vi "Configure Sweep.vi"(0 "VISA resource name":refnum<visa-resource-name>, 1 "Source Type (1: Fixed)":i32(ring)=1 items=["Arbitrary", "Fixed", "Sweep", "List"], 2 "Sweep Output Type (0: Linear Single)":i32(ring) items=["Linear Single", "Linear Double"], 5 "Channel (1: Channel 1)":i32(ring)=1 items=["Channel 1"=1, "Channel 2"=2], 7 "Sweep Stop (0 V)":dbl, 9 "Sweep Start (0 V)":dbl, 11 "error in (no error)":errorcluster, 12 "Sweep Step Number (1)":i32=1) -> (4 "VISA resource name out":refnum<visa-resource-name>, 15 "error out":errorcluster)   [LabVIEW 2012, in "Keysight B2980 Series.lvlib"]
doc: "Configures sweep for measurement and source.\n\n<b>Note(s):</b>\nThis VI is only applicable for model B2985A and B2987A."
uses:
  Keysight B2980 Series.lvlib
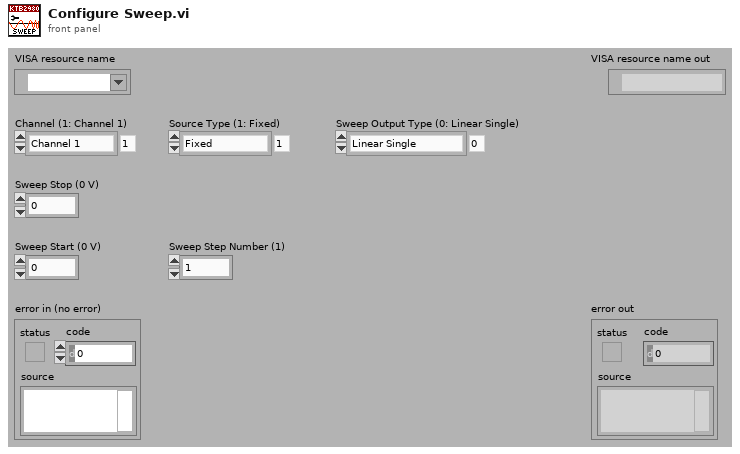
[diagram p1: front panel]
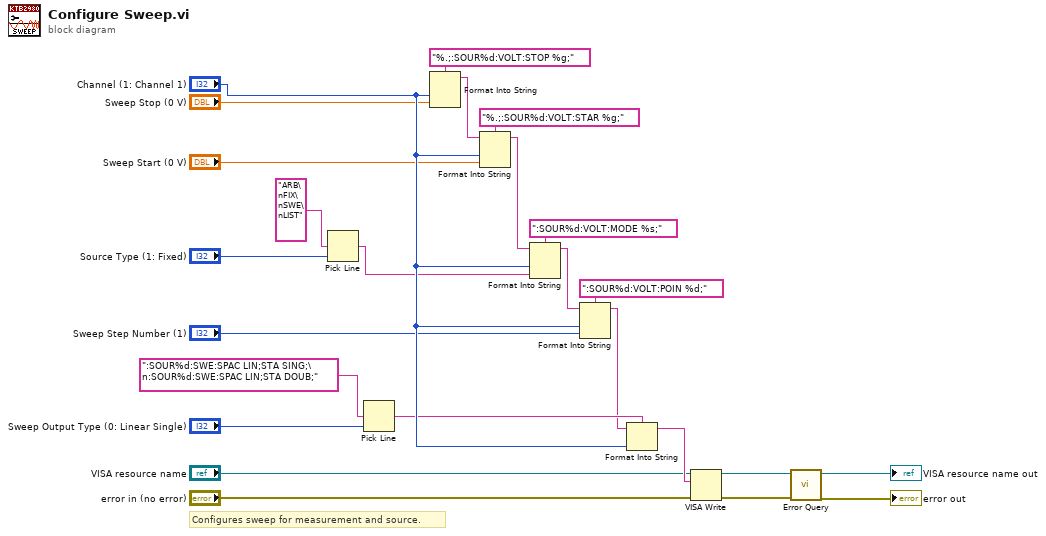
[diagram p0: block diagram]
diagram:
  # "Configures sweep for measurement and source."
  n1 = Pick Line(multi-line string="ARB\nFIX\nSWE\nLIST", line index="Source Type (1: Fixed)") -> (output string=w15:string)  [unwired: 1 out]
  n2 = Pick Line(multi-line string=":SOUR%d:SWE:SPAC LIN;STA SING;\n:SOUR%d:SWE:SPAC LIN;STA DOUB;", line index="Sweep Output Type (0: Linear Single)") -> (output string=w2:string)  [unwired: 1 out]
  n3 = Format Into String(format string="%.;:SOUR%d:VOLT:STOP %g;", "Channel (1: Channel 1)", "Sweep Stop (0 V)") -> (resulting string=w22:string)  [unwired: 2 in, 1 out]
  n4 = Format Into String(format string="%.;:SOUR%d:VOLT:STAR %g;", initial string=w22, "Channel (1: Channel 1)", "Sweep Start (0 V)") -> (resulting string=w17:string)  [unwired: 1 in, 1 out]
  n5 = Format Into String(format string=":SOUR%d:VOLT:MODE %s;", initial string=w17, "Channel (1: Channel 1)", w15) -> (resulting string=w14:string)  [unwired: 1 in, 1 out]
  n6 = Format Into String(format string=":SOUR%d:VOLT:POIN %d;", initial string=w14, "Channel (1: Channel 1)", "Sweep Step Number (1)") -> (resulting string=w1:string)  [unwired: 1 in, 1 out]
  n7 = Format Into String(format string=w2, initial string=w1, "Channel (1: Channel 1)") -> (resulting string=w11:string)  [unwired: 1 in, 1 out]
  n8 = VISA Write(VISA resource name="VISA resource name", write buffer=w11, error in (no error)="error in (no error)") -> (VISA resource name out=w8:refnum<visa-resource-name>, error out=w7:errorcluster)  [unwired: 1 out]
  n9 = call "Error Query.vi"("error in (no error)"=w7, "VISA resource name"=w8) -> ("error out"=→"error out":errorcluster, "VISA resource name out"=→"VISA resource name out":refnum<visa-resource-name>)  [unwired: 8 out]
